vi "CreatePath&FileName.vi"(0 "FileName":string, 4 "Measurement type":T1(ring), 5 "Temp_K":dbl, 6 "AcqTime_ms":dbl, 7 "CenterWL_nm":dbl, 8 "ExcPow_uW":dbl) -> (1 "MeasurementGroupName":string, 2 "DatasetName":string, 3 "File path":path=path "Cluster Attributes.hdf5")   [LabVIEW 2019]
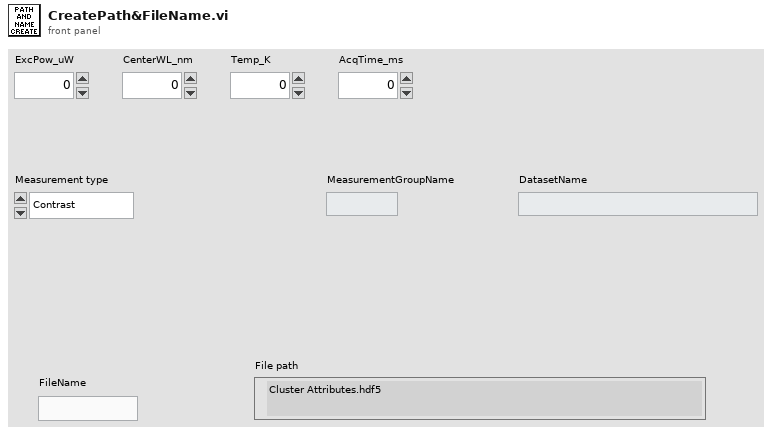
[diagram p1: front panel]
types:
  T1 = enum16{"Contrast", "XY Intensity Map", "Polarisation", "Spectrum"}
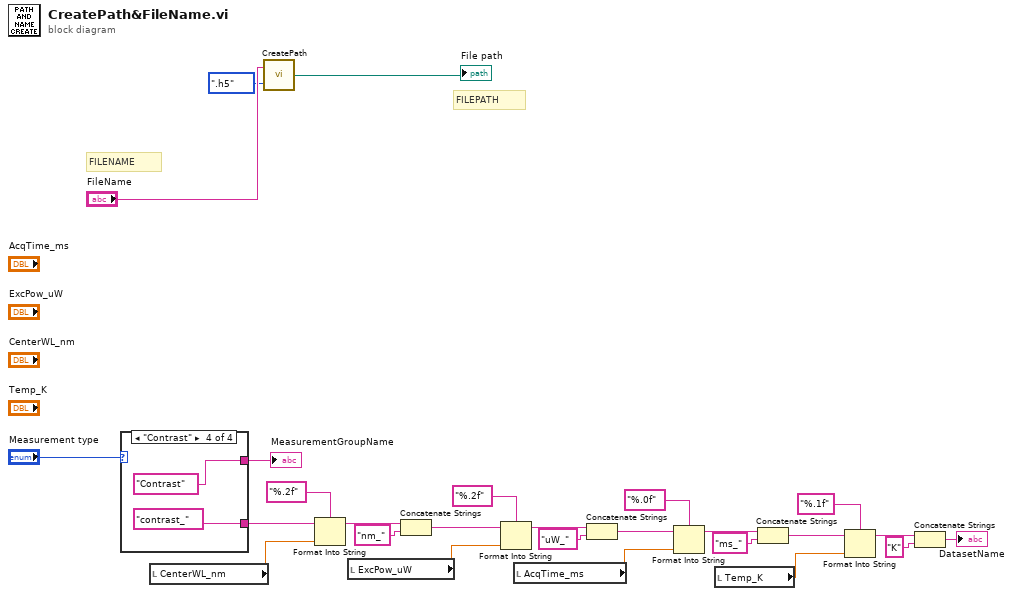
[diagram p0: block diagram]
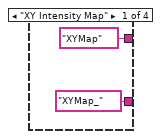
[diagram p2: hidden frame]
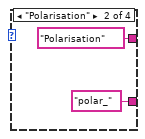
[diagram p3: hidden frame]
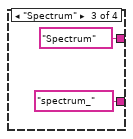
[diagram p4: hidden frame]
diagram:
  # "FILEPATH"
  # "FILENAME"
  n1 = case shown="\"Contrast\"" "Measurement type" {
    tunnel: ["XYMap" "Polarisation" "Spectrum" "Contrast"] -> w25
    tunnel: ["XYMap_" "polar_" "spectrum_" "contrast_"] -> w5
    frame "XY Intensity Map" {
    }
    frame "Polarisation" {
    }
    frame "Spectrum" {
    }
    frame "Contrast" {
    }
  }
  "MeasurementGroupName" <- w25
  n2 = local read "CenterWL_nm"() -> (w14:dbl)
  n3 = call "CreatePath.vi"("filetype"=enum16{".h5", ".txt"}.".h5", "FileName"="FileName") -> ("File path"=→"File path":path)
  n4 = Format Into String(format string="%.2f", initial string=w5, w14) -> (resulting string=w18:string)  [unwired: 1 in, 1 out]
  n5 = local read "ExcPow_uW"() -> (w15:dbl)
  n6 = Concatenate Strings(w18, "nm_") -> (w19:string)
  n7 = Format Into String(format string="%.2f", initial string=w19, w15) -> (resulting string=w20:string)  [unwired: 1 in, 1 out]
  n8 = local read "AcqTime_ms"() -> (w16:dbl)
  n9 = Concatenate Strings(w20, "uW_") -> (w21:string)
  n10 = Format Into String(format string="%.0f", initial string=w21, w16) -> (resulting string=w22:string)  [unwired: 1 in, 1 out]
  n11 = local read "Temp_K"() -> (w17:dbl)
  n12 = Concatenate Strings(w22, "ms_") -> (w23:string)
  n13 = Format Into String(format string="%.1f", initial string=w23, w17) -> (resulting string=w24:string)  [unwired: 1 in, 1 out]
  n14 = Concatenate Strings(w24, "K") -> (→"DatasetName":string)
